vi "Daimler FPGA Main.vi"() -> ()   [LabVIEW 2018]
doc: "This VI reads all analogue data channels available at the fastest rate supported by the respective hardware and updates a memory address for when each measurement is available.\n\nAt a rate defined by the fastest module (NI 9237 - default of 12.5kHz) this memory is read, combined with the measurements from the 9237 module and written to the FIFO for communication to the RT machine.\n\nThe NI 9237 modeul therefore defines the nominal sampling rate of the system (with slower channels over-sampled).\n\nA time channel (in uSec) is provided with 0 referenced from the first acquisition of the NI 9237 module"
uses:
  <vilib>/LabVIEW Targets/FPGA/cRIO/shared/nicrio_ModuleControls/nicrio_cRIO-9237_DataRatesRing.ctl
  <vilib>/rvi/Emulation/niFpgaGetClockAttributes.vi
  <vilib>/rvi/Emulation/niFpgaSctlEmulationGetInTimedLoop.vi
  <vilib>/rvi/Emulation/niFpgaEmulationReportErrorSimple.vi
  <vilib>/rvi/eio/common/nirviEmuTemplatePropertySet_noerrors.vi
  <vilib>/rvi/eio/common/nirviEmuTemplateMethod_errors.vi
  <vilib>/rvi/Memory/Memory_Emulation/nirvimemoryFastEmulation.vi
  <vilib>/rvi/Memory/Memory_Emulation/nirvimemoryEmulation.vi
  <vilib>/rvi/Emulation/niFpgaEmulationIsFPGAContextNoSignature.vi
  <vilib>/rvi/DataTransferAndStorage/Container/Common/niFpgaContainerGetUniqueNameForEmu.vi
  <vilib>/rvi/Emulation/niFpgaProcessEmulError.vi
  <vilib>/rvi/errors/nirviReportUnexpectedCaseInternalError (U32).vi
  <vilib>/rvi/Emulation/niFpgaCriticalErrorInLSC.vi
  <vilib>/eio/EIOPropertyNode/EIOPropertyNode.xnode
  <vilib>/eio/EIONode/EIONode.xnode
  <vilib>/rvi/DataTransferAndStorage/Container/XNode/niFpgaContainer.xnode
  <vilib>/eio/EIOMethodNode/EIOMethodNode.xnode
  <vilib>/rvi/eio/common/nirviEmuTemplatePropertyGet_errors.vi
  <vilib>/rvi/eio/common/nirviEmuTemplatePropertyGet_noerrors.vi
  <vilib>/rvi/eio/common/nirviEmuTemplatePropertySet_errors.vi
panel:
  out "pointsWritten":u16=10000
  in  "dataPoints":u16=10000
  in  "stream":bool
  in  "Data Rate":T1=1 items=["50.000 kS/s (NI 9237)"=1, "25.000 kS/s (NI 9237)"=2, "16.667 kS/s (NI 9237)"=3, "12.500 kS/s (NI 9237)"=4, "10.000 kS/s (NI 9237)"=5, "8.333 kS/s (NI 9237)"=6, "7.143 kS/s (NI 9237)"=7, "6.250 kS/s (NI 9237)"=8, "5.556 kS/s (NI 9237)"=9, "5.000 kS/s (NI 9237)"=10, "4.545 kS/s (NI 9237)"=11, "4.167 kS/s (NI 9237)"=12, "3.846 kS/s (NI 9237)"=13, "3.571 kS/s (NI 9237)"=14, "3.333 kS/s (NI 9237)"=15, "3.125 kS/s (NI 9237)"=16, "2.941 kS/s (NI 9237)"=17, "2.778 kS/s (NI 9237)"=18, "2.632 kS/s (NI 9237)"=19, "2.500 kS/s (NI 9237)"=20, "2.381 kS/s (NI 9237)"=21, "2.273 kS/s (NI 9237)"=22, "2.174 kS/s (NI 9237)"=23, "2.083 kS/s (NI 9237)"=24, "2.000 kS/s (NI 9237)"=25, "1.923 kS/s (NI 9237)"=26, "1.852 kS/s (NI 9237)"=27, "1.786 kS/s (NI 9237)"=28, "1.724 kS/s (NI 9237)"=29, "1.667 kS/s (NI 9237)"=30, "1.613 kS/s (NI 9237)"=31]
  out "Total channel count":u32=61
  out "timestamp":u32
  in  "Voltage Out":fxp<+/-,20,5>[](array[numeric])=[0.0, 0.0, 0.0, 0.0]
  in  "Update Outputs":bool
  in  "Mod 8":bool[](array[boolean])=[FALSE, FALSE, FALSE, FALSE, FALSE, FALSE, FALSE, FALSE]
  in  "Stop acquire":bool
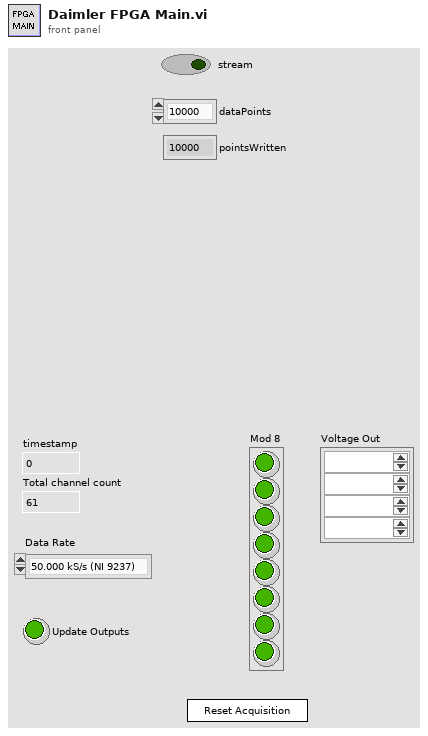
[diagram p1: front panel]
types:
  T1 = typedef "nicrio_cRIO-9237_DataRatesRing.ctl" = u8
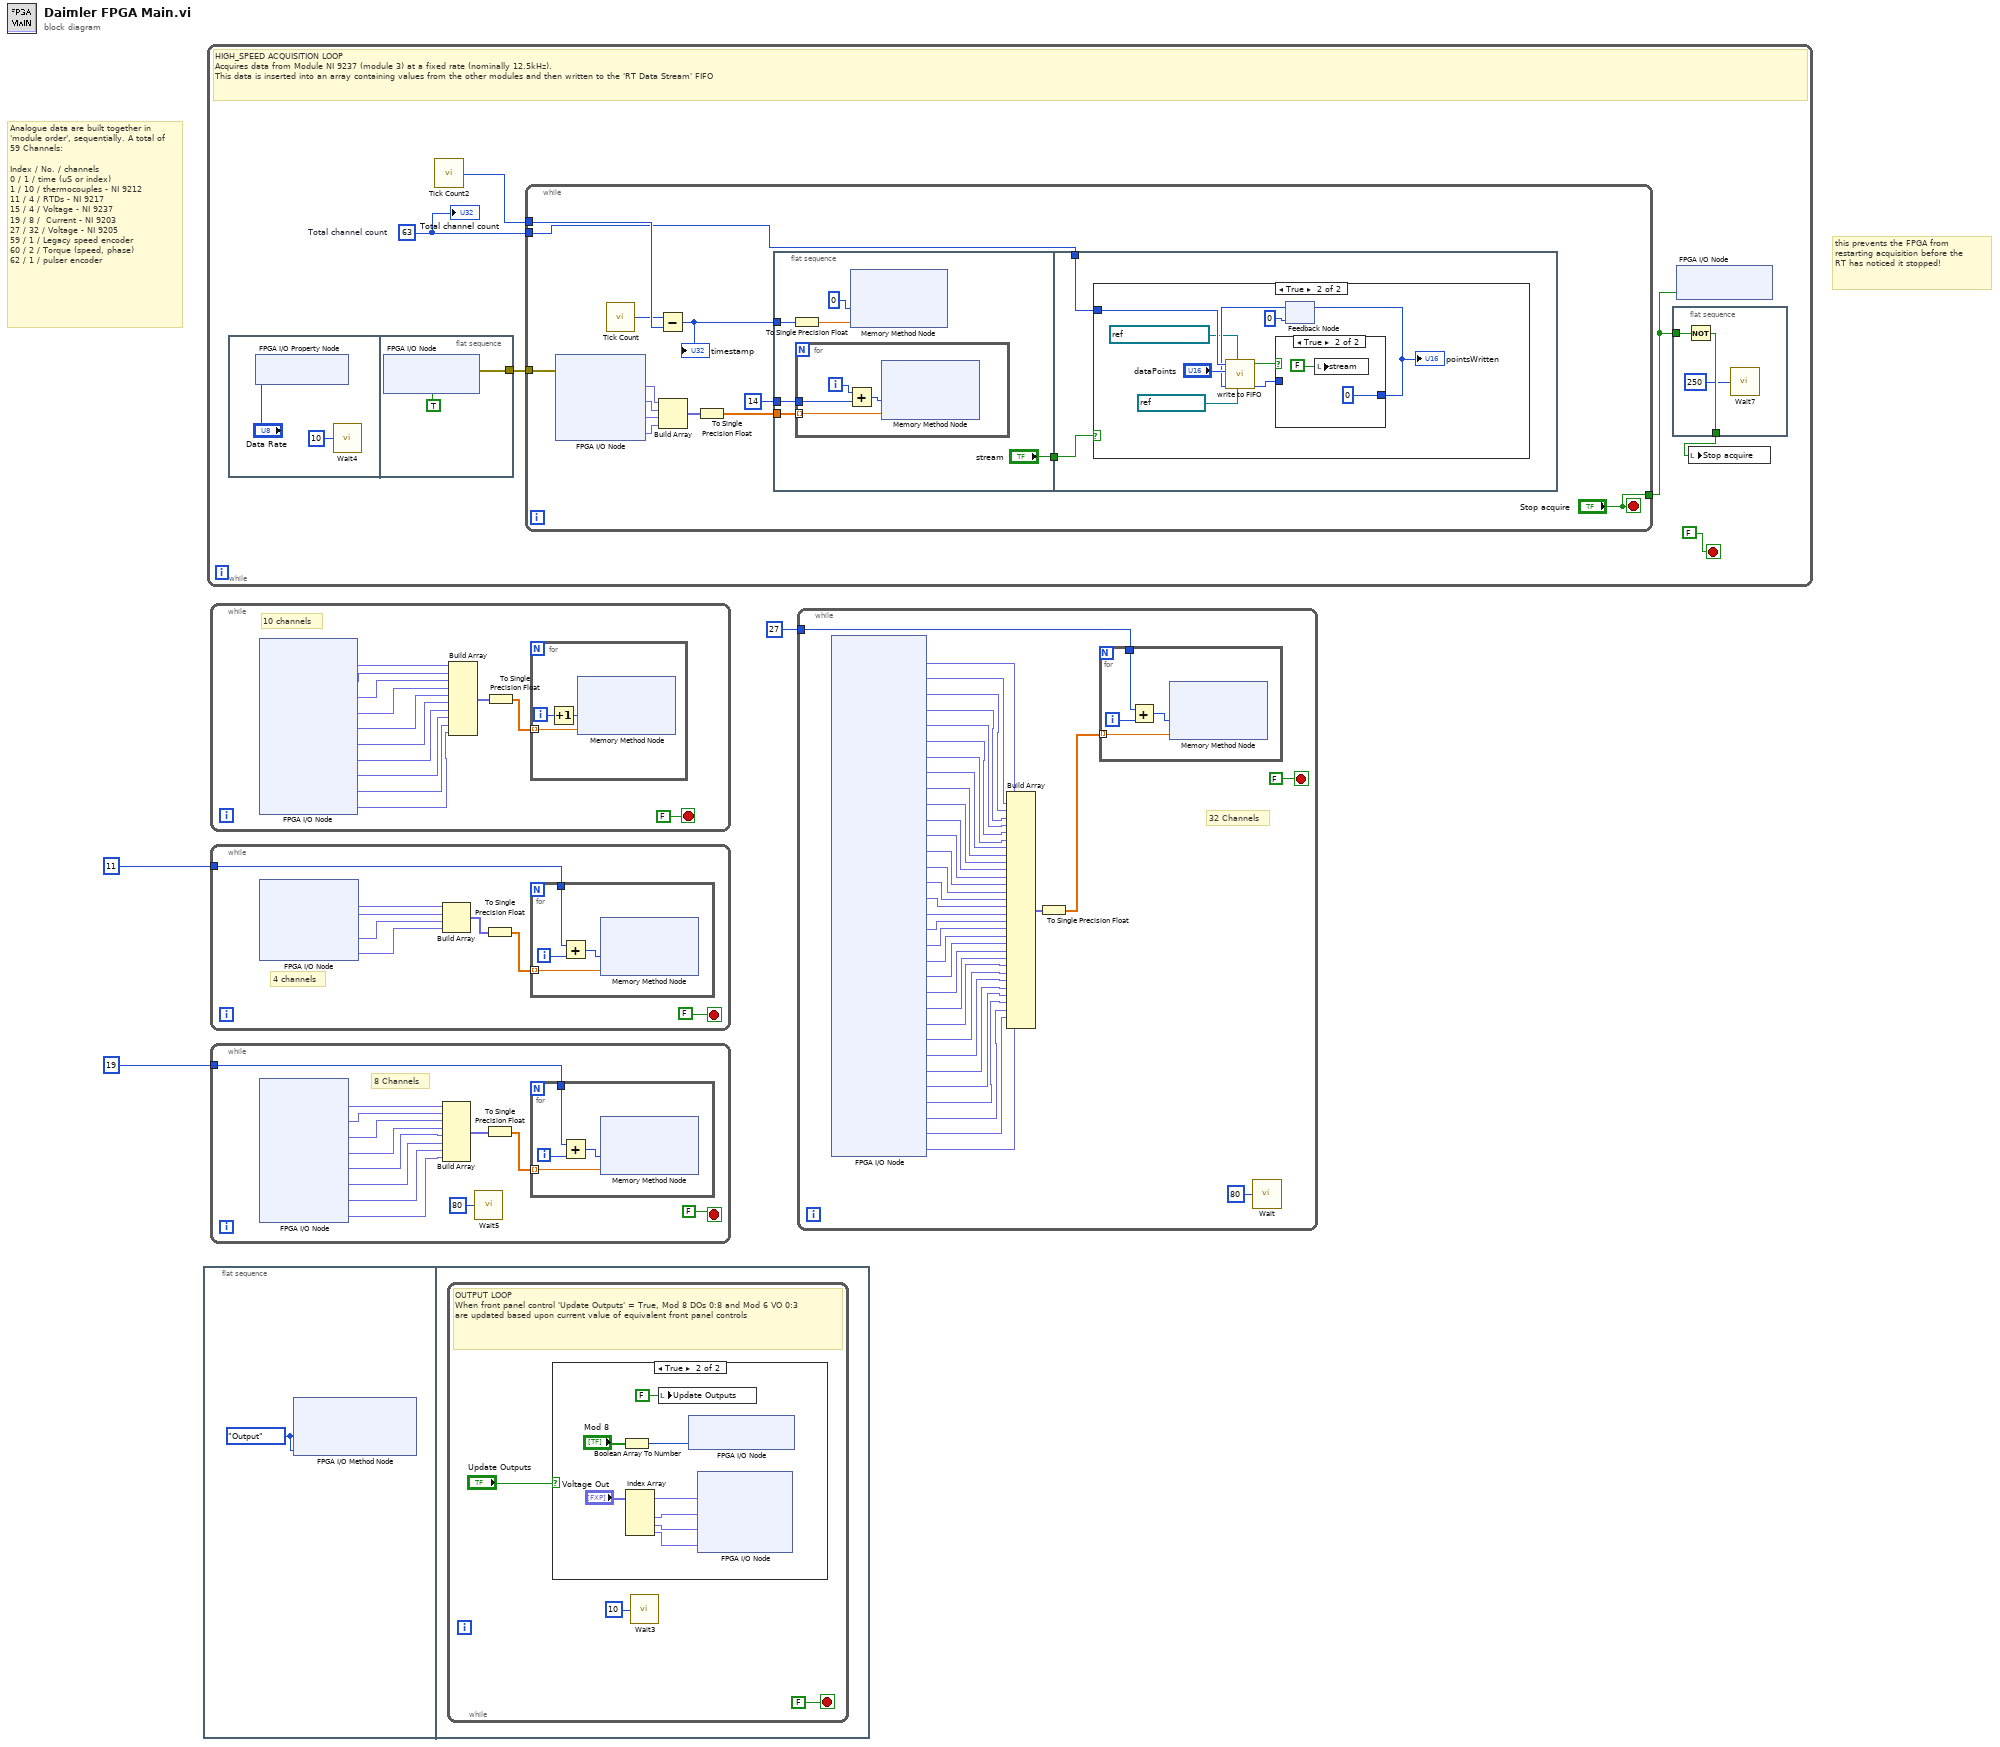
[diagram p0: block diagram]
diagram:
  # "this prevents the FPGA from restarting acquisition before the RT has noticed it stopped!"
  # "Analogue data are built together in 'module order', sequentially. A total of 59 Channels:\n\nIndex / No. / channels\n0 / 1 / time (uS or index)\n1 / 10 / thermocouples - NI 9212\n11 / 4 / RTDs - NI 9217\n15 / 4 / Voltage - NI 9237\n19 / 8 /  Current - NI 9203\n27 / 32 / Voltage - NI 9205\n59 / 1 / Legacy speed encoder\n60 / 2 / Torque (speed, phase)\n62 / 1 / pulser encoder"
  n1 = flat-sequence {
    frame #0 {
      w4 = enum8{"No Change", "Input", "Output"}."Output" ("DIO 7:4")
      n2 = xnode "FPGA I/O Method Node"("DIO 7:4"=w4, "DIO 3:0"=w4) -> ()  [unwired: 1 in, 1 out]
    }
    frame #1 {
      n3 = while {
        stop <- FALSE stop-if-true
        # "OUTPUT LOOP\nWhen front panel control 'Update Outputs' = True, Mod 8 DOs 0:8 and Mod 6 VO 0:3 are updated based upon current value of equivalent front panel controls"
        n4 = case shown="True" "Update Outputs" {
          frame False {
          }
          frame True {
            n5 = Boolean Array To Number(Boolean array="Mod 8") -> (number=w14:u8)
            n6 = Index Array(array="Voltage Out") -> (element #1=w12:fxp<+/-,20,5>, element #2=w11:fxp<+/-,20,5>, element #3=w10:fxp<+/-,20,5>, element #4=w9:fxp<+/-,20,5>)  [unwired: 4 in]
            n7 = local write "Update Outputs"(FALSE ("Update Outputs")) -> ()
            n8 = xnode "FPGA I/O Node"("Mod8/DIO7:0"=w14) -> ()  [unwired: 1 in, 1 out]
            n9 = xnode "FPGA I/O Node"("Mod6/AO0"=w12, "Mod6/AO1"=w11, "Mod6/AO2"=w10, "Mod6/AO3"=w9) -> ()  [unwired: 4 in, 4 out]
          }
        }
        n10 = call "Wait3"("Count(uSec)"=u16 10 ("Count(Ticks)")) -> ()  [unwired: 1 out]
      }
    }
  }
  n11 = while {
    stop <- FALSE stop-if-true
    w19 = u32 63  # Total channel count
    # "HIGH_SPEED ACQUISITION LOOP\nAcquires data from Module NI 9237 (module 3) at a fixed rate (nominally 12.5kHz).\nThis data is inserted into an array containing values from the other modules and then written to the 'RT Data Stream' FIFO"
    n12 = flat-sequence {
      tunnel: [w28] -> w20
      frame #0 {
        n13 = xnode "FPGA I/O Property Node"("Data Rate"="Data Rate") -> ()  [unwired: 1 in, 1 out]
        n14 = call "Wait4"("Count(mSec)"=u16 10) -> ()  [unwired: 1 out]
      }
      frame #1 {
        n15 = xnode "FPGA I/O Node"("Mod3/Start"=TRUE) -> ("error out"=w28:errorcluster)  [unwired: 2 in, 1 out]
      }
    }
    n16 = call "Tick Count2"() -> ("Tick Count(uSec)"=w21:u32)
    n17 = while {
      tunnel: ["Stop acquire"] -> w18
      tunnel: w20 -> [w42]
      tunnel: w19 -> [w30]
      tunnel: w21 -> [w36]
      stop <- "Stop acquire" stop-if-true
      n18 = xnode "FPGA I/O Node"("error in"=w42) -> ("Mod3/AI0"=w41:fxp<+/-,24,-4>, "Mod3/AI1"=w40:fxp<+/-,24,-4>, "Mod3/AI2"=w39:fxp<+/-,24,-4>, "Mod3/AI3"=w38:fxp<+/-,24,-4>)  [unwired: 4 in, 5 out]
      n19 = call "Tick Count"() -> ("Tick Count(uSec)"=w35:u32)
      n20 = Subtract(x=w35, y=w36) -> (x-y=w32:u32)
      "timestamp" <- w32
      n21 = Build Array(w41, w40, w39, w38) -> (w37:fxp<+/-,24,-4>[])
      n22 = To Single Precision Float(number=w37) -> (single precision float=w34:sgl[])
      n23 = flat-sequence {
        tunnel: w34 -> [w48]
        tunnel: 14 ("index") -> [w47]
        tunnel: w32 -> [w45]
        tunnel: ["stream"] -> w31
        tunnel: w31 -> [w54]
        tunnel: w30 -> [w53]
        frame #0 {
          n24 = To Single Precision Float(number=w45) -> (single precision float=w46:sgl)
          n25 = for {
            tunnel: w48 -> [w52] mode=indexing
            tunnel: w47 -> [w51]
            i -> [w49]
            n26 = Add(x=w49, y=w51) -> (x+y=w50:i32)
            n27 = xnode ("Memory Method Node")("Address"=w50, "Data"=w52) -> ()  [unwired: 1 in, 1 out]
          }
          n28 = xnode ("Memory Method Node")("Address"=u32 0, "Data"=w46) -> ()  [unwired: 1 in, 1 out]
        }
        frame #1 {
          n29 = case shown="True" w54 {
            tunnel: w53 -> [_ w63]
            frame False {
            }
            frame True {
              n30 = feedback #1(u16 0 ("pointsWritten")) -> (w60:u16)
              n31 = call "write to FIFO.vi"("Memory In"=refnum<k21> "Memory", "FIFO In"=refnum<k21> "RT Data Stream", "points_written"=w60, "dataPoints"="dataPoints", "channelCount"=w63) -> ("pointsWritten"=w58:u16, "done"=w62:bool)  [unwired: 5 in]
              n32 = case shown="True" w62 {
                tunnel: [w64 u16 0 ("pointsWritten")] -> w57
                tunnel: w58 -> [w64 _]
                frame False {
                }
                frame True {
                  n33 = local write "stream"(FALSE ("stream")) -> ()
                }
              }
              "pointsWritten" <- w57
              n34 = feedback-in #1(w57) -> ()
            }
          }
        }
      }
    }
    n35 = flat-sequence {
      tunnel: w18 -> [w24]
      tunnel: [w23] -> w16
      frame #0 {
        n36 = Not(x=w24) -> (.not. x?=w23:bool)
        n37 = call "Wait7"("Count(mSec)"=u8 250) -> ()  [unwired: 1 out]
      }
    }
    n38 = xnode "FPGA I/O Node"("Mod3/Stop"=w18) -> ()  [unwired: 1 in, 1 out]
    n39 = local write "Stop acquire"(w16) -> ()
    "Total channel count" <- w19
  }
  n40 = while {
    stop <- FALSE stop-if-true
    # "10 channels"
    n41 = xnode "FPGA I/O Node"() -> ("Mod1/TC0"=w79:fxp<+/-,24,-2>, "Mod1/TC1"=w78:fxp<+/-,24,-2>, "Mod1/TC2"=w77:fxp<+/-,24,-2>, "Mod1/TC3"=w76:fxp<+/-,24,-2>, "Mod1/TC4"=w75:fxp<+/-,24,-2>, "Mod1/TC5"=w74:fxp<+/-,24,-2>, "Mod1/TC6"=w73:fxp<+/-,24,-2>, "Mod1/TC7"=w72:fxp<+/-,24,-2>, "Mod1/CJC0"=w69:fxp<+/-,24,-2>, "Mod1/CJC1"=w68:fxp<+/-,24,-2>)  [unwired: 10 in, 10 out]
    n42 = Build Array(w79, w78, w77, w76, w75, w74, w73, w72, w69, w68) -> (w71:fxp<+/-,24,-2>[])
    n43 = To Single Precision Float(number=w71) -> (single precision float=w70:sgl[])
    n44 = for {
      tunnel: w70 -> [w82] mode=indexing
      i -> [w81]
      n45 = Increment(x=w81) -> (x+1=w80:i32)
      n46 = xnode ("Memory Method Node")("Address"=w80, "Data"=w82) -> ()  [unwired: 1 in, 1 out]
    }
  }
  n47 = while {
    tunnel: 11 ("Numeric") -> [w84]
    stop <- FALSE stop-if-true
    # "4 channels"
    n48 = xnode "FPGA I/O Node"() -> ("Mod2/RTD0"=w90:fxp<+/-,24,10>, "Mod2/RTD1"=w89:fxp<+/-,24,10>, "Mod2/RTD2"=w88:fxp<+/-,24,10>, "Mod2/RTD3"=w85:fxp<+/-,24,10>)  [unwired: 4 in, 4 out]
    n49 = Build Array(w90, w89, w88, w85) -> (w87:fxp<+/-,24,10>[])
    n50 = To Single Precision Float(number=w87) -> (single precision float=w86:sgl[])
    n51 = for {
      tunnel: w86 -> [w94] mode=indexing
      tunnel: w84 -> [w91]
      i -> [w93]
      n52 = Add(x=w91, y=w93) -> (x+y=w92:i32)
      n53 = xnode ("Memory Method Node")("Address"=w92, "Data"=w94) -> ()  [unwired: 1 in, 1 out]
    }
  }
  n54 = while {
    tunnel: 19 ("Numeric") -> [w101]
    stop <- FALSE stop-if-true
    # "8 Channels"
    n55 = xnode "FPGA I/O Node"() -> ("Mod4/AI0"=w107:fxp<+/-,21,-4>, "Mod4/AI1"=w106:fxp<+/-,21,-4>, "Mod4/AI2"=w105:fxp<+/-,21,-4>, "Mod4/AI3"=w102:fxp<+/-,21,-4>, "Mod4/AI4"=w100:fxp<+/-,21,-4>, "Mod4/AI5"=w99:fxp<+/-,21,-4>, "Mod4/AI6"=w98:fxp<+/-,21,-4>, "Mod4/AI7"=w97:fxp<+/-,21,-4>)  [unwired: 8 in, 8 out]
    n56 = Build Array(w107, w106, w105, w102, w100, w99, w98, w97) -> (w104:fxp<+/-,21,-4>[])
    n57 = call "Wait5"("Count(uSec)"=u8 80) -> ()  [unwired: 1 out]
    n58 = To Single Precision Float(number=w104) -> (single precision float=w103:sgl[])
    n59 = for {
      tunnel: w103 -> [w111] mode=indexing
      tunnel: w101 -> [w108]
      i -> [w110]
      n60 = Add(x=w108, y=w110) -> (x+y=w109:i32)
      n61 = xnode ("Memory Method Node")("Address"=w109, "Data"=w111) -> ()  [unwired: 1 in, 1 out]
    }
  }
  n62 = while {
    tunnel: 27 ("Numeric") -> [w147]
    stop <- FALSE stop-if-true
    # "32 Channels"
    n63 = xnode "FPGA I/O Node"() -> ("Mod5/AI0"=w115:fxp<+/-,26,5>, "Mod5/AI1"=w116:fxp<+/-,26,5>, "Mod5/AI2"=w117:fxp<+/-,26,5>, "Mod5/AI3"=w118:fxp<+/-,26,5>, "Mod5/AI4"=w119:fxp<+/-,26,5>, "Mod5/AI5"=w120:fxp<+/-,26,5>, "Mod5/AI6"=w121:fxp<+/-,26,5>, "Mod5/AI7"=w122:fxp<+/-,26,5>, "Mod5/AI8"=w146:fxp<+/-,26,5>, "Mod5/AI9"=w145:fxp<+/-,26,5>, "Mod5/AI10"=w144:fxp<+/-,26,5>, "Mod5/AI11"=w143:fxp<+/-,26,5>, "Mod5/AI12"=w142:fxp<+/-,26,5>, "Mod5/AI13"=w141:fxp<+/-,26,5>, "Mod5/AI14"=w140:fxp<+/-,26,5>, "Mod5/AI15"=w139:fxp<+/-,26,5>, "Mod5/AI16"=w138:fxp<+/-,26,5>, "Mod5/AI17"=w137:fxp<+/-,26,5>, "Mod5/AI18"=w136:fxp<+/-,26,5>, "Mod5/AI19"=w135:fxp<+/-,26,5>, "Mod5/AI20"=w134:fxp<+/-,26,5>, "Mod5/AI21"=w133:fxp<+/-,26,5>, "Mod5/AI22"=w132:fxp<+/-,26,5>, "Mod5/AI23"=w131:fxp<+/-,26,5>, "Mod5/AI24"=w130:fxp<+/-,26,5>, "Mod5/AI25"=w129:fxp<+/-,26,5>, "Mod5/AI26"=w128:fxp<+/-,26,5>, "Mod5/AI27"=w127:fxp<+/-,26,5>, "Mod5/AI28"=w126:fxp<+/-,26,5>, "Mod5/AI29"=w125:fxp<+/-,26,5>, "Mod5/AI30"=w124:fxp<+/-,26,5>, "Mod5/AI31"=w123:fxp<+/-,26,5>)  [unwired: 32 in, 32 out]
    n64 = Build Array(w115, w116, w117, w118, w119, w120, w121, w122, w146, w145, w144, w143, w142, w141, w140, w139, w138, w137, w136, w135, w134, w133, w132, w131, w130, w129, w128, w127, w126, w125, w124, w123) -> (w148:fxp<+/-,26,5>[])
    n65 = To Single Precision Float(number=w148) -> (single precision float=w114:sgl[])
    n66 = for {
      tunnel: w114 -> [w152] mode=indexing
      tunnel: w147 -> [w149]
      i -> [w151]
      n67 = Add(x=w149, y=w151) -> (x+y=w150:i32)
      n68 = xnode ("Memory Method Node")("Address"=w150, "Data"=w152) -> ()  [unwired: 1 in, 1 out]
    }
    n69 = call "Wait"("Count(uSec)"=u8 80) -> ()  [unwired: 1 out]
  }
